vi "Set_Sub_Collection.vi"(8 "error in (no error)":errorcluster caption="entrée d'erreur (pas d'erreur)", 11 "Firebase PCBA en entrée":refnum<class "Firebase Altyor.lvclass">) -> (0 "error out":errorcluster caption="sortie d'erreur", 3 "Firebase PCBA en sortie":refnum<class "Firebase Altyor.lvclass">)   [LabVIEW 2020, in "Library Instrument & Equipement.lvlib" / "Library FireBase.lvlib" / "Firebase Altyor.lvclass"]
doc: "Create New document\nPlease initialise the following values\n - Name BDD\n - Document of test sequence\n - API Key"
uses:
  Firebase Altyor.lvclass
  C:/Users/ngarcin/OneDrive - Altyor/Standard TB/Class/Firebase/Source/Firebase Driver/Firebase Driver.lvclass
  Firebase Altyor.lvclass/Firebase Altyor.ctl
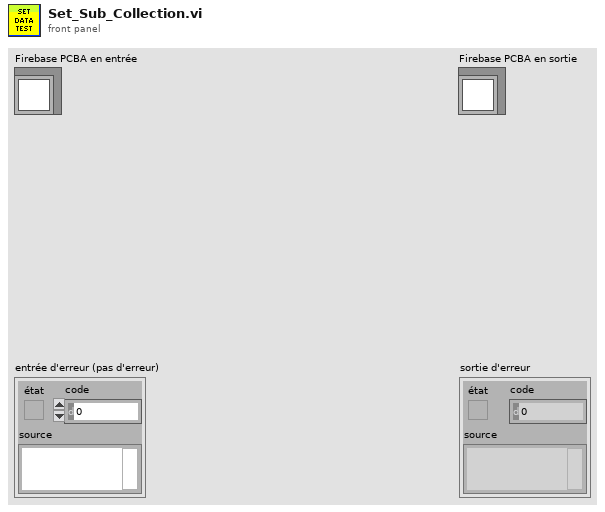
[diagram p1: front panel]
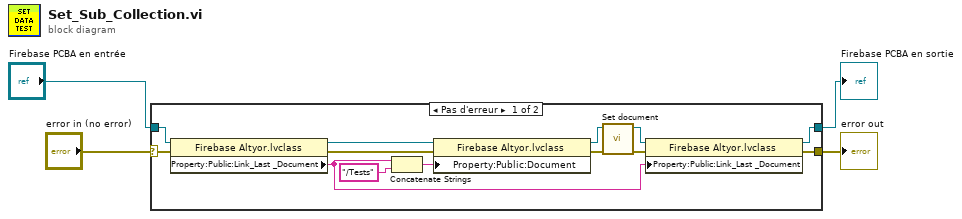
[diagram p0: block diagram]
diagram:
  n1 = case shown="Pas d'erreur" "error in (no error)" {
    selector: "error in (no error)" -> [w16 w19]
    tunnel: [w9 w19] -> w3
    tunnel: [w5 w18] -> w1
    tunnel: "Firebase PCBA en entrée" -> [w13 w18]
    frame No Error {
      n2 = property class="Firebase Altyor.lvclass"(reference=w13, error in=w16) -> (reference out=w15:refnum<class "Firebase Altyor.lvclass">, error out=w14:errorcluster, "Property:Public:Link_Last _Document"=w8:string)
      n3 = Concatenate Strings(w8, "/Tests" ("chaîne")) -> (w12:string)
      n4 = property class="Firebase Altyor.lvclass"(reference=w15, error in=w14, "Property:Public:Document"=w12) -> (reference out=w7:refnum<class "Firebase Altyor.lvclass">, error out=w6:errorcluster)
      n5 = call-dynamic "Set document.vi"("error in (no error)"=w6, "Firebase (Default) en entrée"=w7) -> ("error out"=w10:errorcluster, "Firebase (Default) en sortie"=w11:refnum<class "Firebase Altyor.lvclass">)  [unwired: 8 in]
      n6 = property class="Firebase Altyor.lvclass"(reference=w11, error in=w10, "Property:Public:Link_Last _Document"=w8) -> (reference out=w5:refnum<class "Firebase Altyor.lvclass">, error out=w9:errorcluster)
    }
    frame Error {
    }
  }
  "error out" <- w3
  "Firebase PCBA en sortie" <- w1
